vi "StartProcessingLoopAsync.vi"(8 "error in (no error)":errorcluster, 10 "navX Class in":refnum<class "navX - Interface.lvclass">, 11 "navX in":refnum<class "navX.lvclass">) -> (0 "error out":errorcluster, 3 "navX out":refnum<class "navX.lvclass">)   [LabVIEW 2015, in "navX Library v3.lvlib" / "navX.lvclass"]
uses:
  navX.lvclass
  navX - Interface/navX - Interface.lvclass
  navX.lvclass/navX.ctl
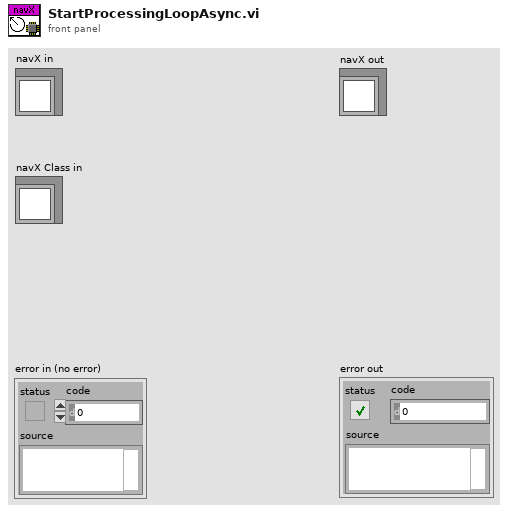
[diagram p1: front panel]
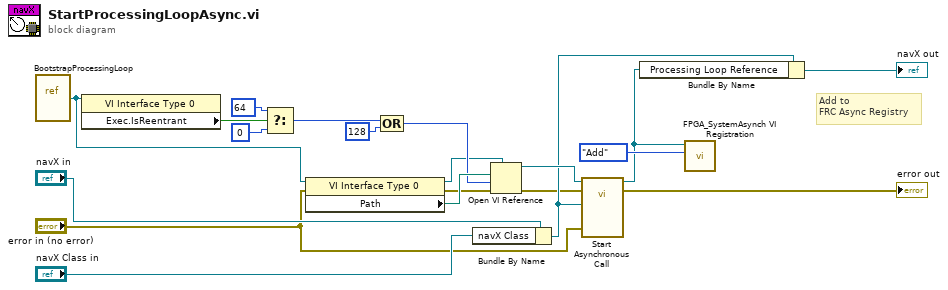
[diagram p0: block diagram]
diagram:
  # "Add to\nFRC Async Registry"
  n1 = vi-ref "BootstrapProcessingLoop.vi"() -> (w6:refnum<vi>)
  n2 = property class="VI Interface Type 0"(reference=w6) -> ("Exec.IsReentrant"=w5:bool)  [unwired: 1 in, 2 out]
  n3 = Select(t=64 ("value"), s=w5, f=0 ("value")) -> (s? t:f=w2:i32)
  n4 = property class="VI Interface Type 0"(reference=w6, error in="error in (no error)") -> (reference out=w7:refnum<vi>, error out=w10:errorcluster, "Path"=w20:path)
  n5 = Compound Arithmetic op=OR(w2, 128 ("value")) -> (w15:i32)
  n6 = Bundle By Name(cluster="navX in", "navX Class"="navX Class in") -> (w12:refnum<class "navX.lvclass">)
  n7 = Open VI Reference(type specifier VI Refnum (for type only)=w7, vi path=w20, options=w15, error in (no error)=w10) -> (vi reference=w19:refnum<vi>, error out=w9:errorcluster)  [unwired: 2 in]
  n8 = call-by-ref "Start Asynchronous Call"(reference=w19, error in=w9, 8:"error in (no error)"="error in (no error)", "navX in"=w12) -> (reference out=w13:refnum<vi>, error out=→"error out":errorcluster)  [unwired: 8 in, 2 out]
  n9 = Bundle By Name(cluster=w12, "Processing Loop Reference"=w13) -> (→"navX out":refnum<class "navX.lvclass">)
  n10 = call <vilib>:"FPGA_SystemAsynch VI Registration.vi"("Operation"=enum16{"Get", "Add", "Remove"}."Add", "VI Refnum"=w13) -> ()  [unwired: 10 out]
